vi "Select Station.vi"(8 "error in (no error)":errorcluster, 10 "FP Frontmost":bool=TRUE, 11 "PLC Sim Controller Actor in":refnum<class "PLC Sim Controller Actor.lvclass">) -> (0 "error out":errorcluster, 3 "PLC Sim Controller Actor out":refnum<class "PLC Sim Controller Actor.lvclass">)   [LabVIEW 2019, in "PLC Sim Controller Actor.lvlib" / "PLC Sim Controller Actor.lvclass"]
uses:
  PLC Sim Controller Actor.lvclass
  PLC Sim Controller Actor.lvclass/PLC Sim Controller Actor.ctl
  Station Actor/Station Actor Messages/FP Frontmost Msg/FP Frontmost Msg.lvclass/FP Frontmost Msg.ctl
  <vilib>/ActorFramework/Message Enqueuer/Message Enqueuer.lvclass/Message Enqueuer.ctl
  <vilib>/ActorFramework/Message Enqueuer/Enqueue.vi
  Station Actor/Station Actor Messages/FP Frontmost Msg/FP Frontmost Msg.lvclass
  C:/Program Files (x86)/National Instruments/LabVIEW 2019/vi.lib/ActorFramework/Message/Message.lvclass
  <vilib>/ActorFramework/Message Priority Queue/Priority Enqueue.vi
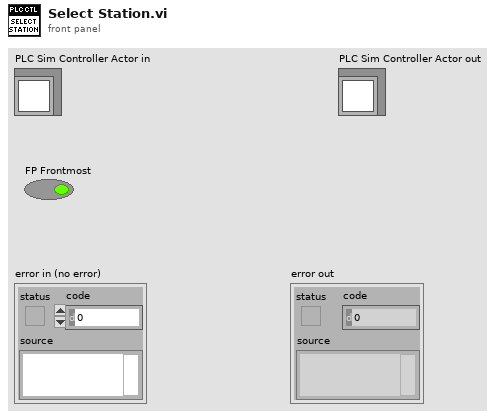
[diagram p1: front panel]
types:
  T1 = map{string, refnum<class "Message Enqueuer.lvclass">}
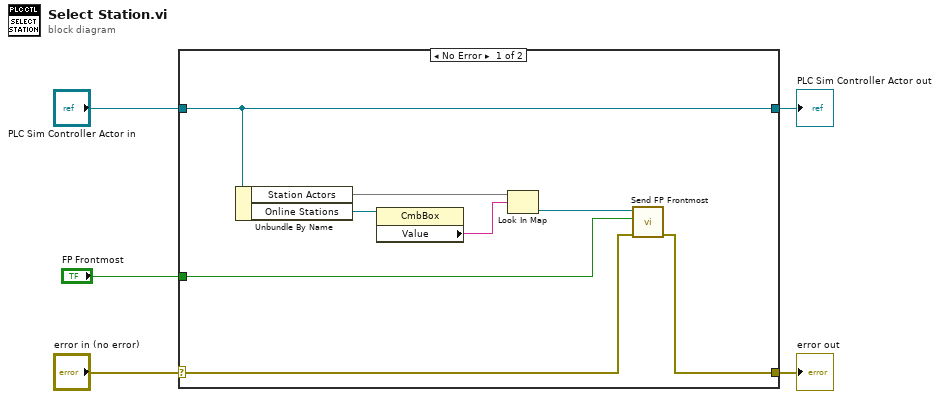
[diagram p0: block diagram]
diagram:
  n1 = case shown="No Error" "error in (no error)" {
    selector: "error in (no error)" -> [w7 w15]
    tunnel: [w6 w15] -> w4
    tunnel: [w10 w14] -> w2
    tunnel: "PLC Sim Controller Actor in" -> [w10 w14]
    tunnel: "FP Frontmost" -> [w8 _]
    frame No Error {
      n2 = Unbundle By Name(w10) -> ("Station Actors"=w11:T1, "Online Stations"=w12:refnum<vi>)
      n3 = property class="CmbBox"(reference=w12) -> ("Value"=w13:string)  [unwired: 1 in, 2 out]
      n4 = Look In Map(map=w11, key=w13) -> (value=w9:refnum<class "Message Enqueuer.lvclass">)  [unwired: 1 in, 1 out]
      n5 = call "Send FP Frontmost.vi"("error in (no error)"=w7, "FP Frontmost"=w8, "Message Enqueuer"=w9) -> ("error out"=w6:errorcluster)  [unwired: 7 in, 1 out]
    }
    frame Error {
    }
  }
  "error out" <- w4
  "PLC Sim Controller Actor out" <- w2
